vi "RTS Read Room CFG.vi"(8 "Error In":errorcluster, 11 "Room CFG File Path":path) -> (0 "error out":errorcluster, 2 "Config Filenames":string[](array[string]), 3 "Search File Path":path)   [LabVIEW 2016]
uses:
  <vilib>/Utility/error.llb/whitespace.ctl
  <vilib>/Utility/file.llb/Read Delimited Spreadsheet (string).vi
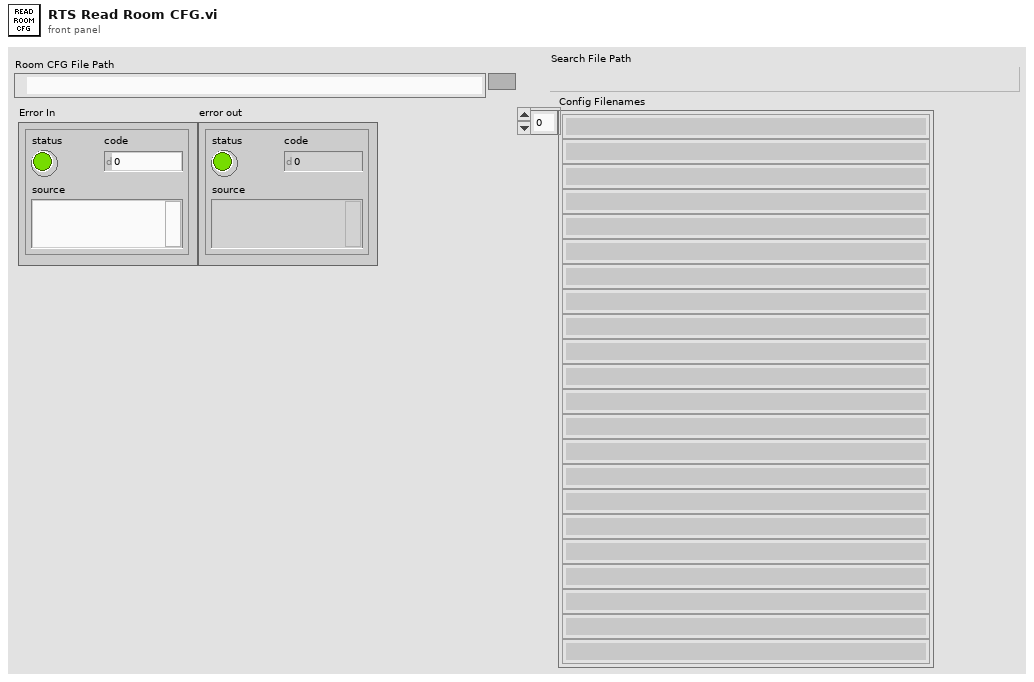
[diagram p1: front panel]
types:
  T1 = typedef "whitespace.ctl" = u16
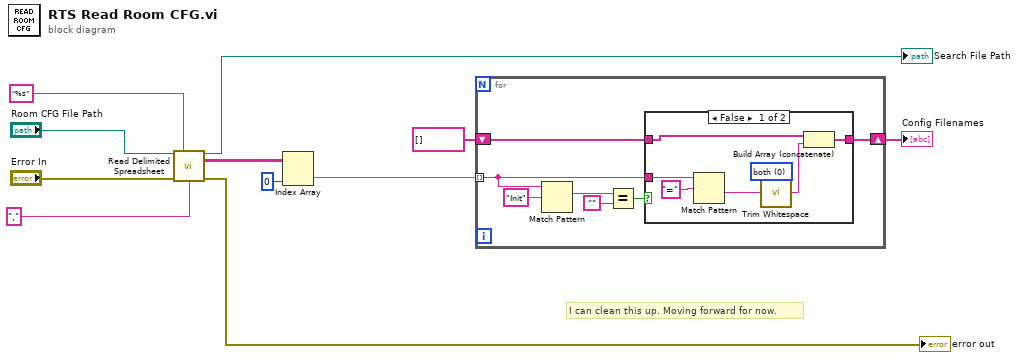
[diagram p0: block diagram]
diagram:
  # "I can clean this up. Moving forward for now."
  n1 = call-poly <vilib>:"Read Delimited Spreadsheet.vi"("file path (dialog if empty)"="Room CFG File Path", "format (%s)"="%s", "error in (no error)"="Error In", "delimiter (\\t)"="," ("delimiter (\\t)")) -> ("new file path (Not A Path if cancelled)"=→"Search File Path":path, "all rows"=w5:string[][], "error out"=→"error out":errorcluster)  [unwired: 6 in, 3 out]
  n2 = Index Array(array=w5, index (col)=0 ("disabled index (col)")) -> (element=w3:string[])  [unwired: 1 in]
  n3 = for {
    tunnel: w3 -> [w12] mode=indexing
    shift-right: [w13] -> w1
    shift-left: string[] [] -> [w14]
    n4 = Match Pattern(string=w12, regular expression="Init") -> (match substring=w17:string)  [unwired: 1 in, 3 out]
    n5 = Equal?(x=w17, y="") -> (x = y?=w15:bool)
    n6 = case shown="False" w15 {
      tunnel: w14 -> [w25 w26]
      tunnel: [w24 w26] -> w13
      tunnel: w12 -> [w23 _]
      frame False {
        w20 = T1 0 items=["both", "start of string", "end of string"] ("location (both)")
        n7 = Match Pattern(string=w23, regular expression="=") -> (after substring=w21:string)  [unwired: 1 in, 3 out]
        n8 = call <vilib>:"Trim Whitespace.vi"("string"=w21, "location (both)"=w20) -> ("trimmed string"=w19:string)
        n9 = Build Array (concatenate)(w25, w19) -> (w24:string[])
      }
      frame True {
      }
    }
  }
  "Config Filenames" <- w1
